vi "UPDATE SETTINGS.vi"(11 "REFERENCES":T1) -> ()   [LabVIEW 2019]
uses:
  Controls/References Cluster.ctl
  Controls/Custom Calendar/Custom Calendar.xctl
  <vilib>/addons/database/Connection.llb/DB Tools Open Connec (String).vi
  <vilib>/addons/database/NI_Database_API.lvlib
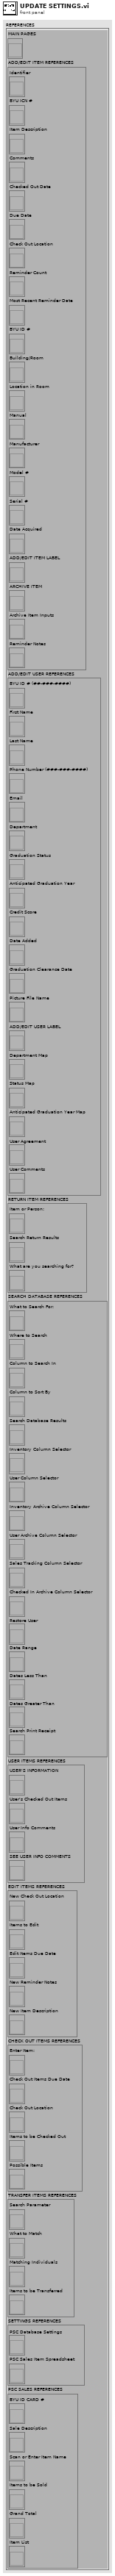
[diagram p1: front panel]
types:
  T1 = typedef "References Cluster.ctl" = cluster{"MAIN PAGES":refnum<vi>, "ADD/EDIT ITEM REFERENCES":cluster{"Identifier":refnum<vi>, "BYU ICN #":refnum<vi>, "Item Description":refnum<vi>, "Comments":refnum<vi>, "Checked Out Date":refnum<vi>, "Due Date":refnum<vi>, "Check Out Location":refnum<vi>, "Reminder Count":refnum<vi>, "Most Recent Reminder Date":refnum<vi>, "BYU ID #":refnum<vi>, "Building/Room":refnum<vi>, "Location in Room":refnum<vi>, "Manual":refnum<vi>, "Manufacturer":refnum<vi>, "Model #":refnum<vi>, "Serial #":refnum<vi>, "Date Acquired":refnum<vi>, "ADD/EDIT ITEM LABEL":refnum<vi>, "ARCHIVE ITEM":refnum<vi>, "Archive Item Inputs":refnum<vi>, "Reminder Notes":refnum<vi>}, "ADD/EDIT USER REFERENCES":cluster{"BYU ID # (##-###-####)":refnum<vi>, "First Name":refnum<vi>, "Last Name":refnum<vi>, "Phone Number (###-###-####)":refnum<vi>, "Email":refnum<vi>, "Department":refnum<vi>, "Graduation Status":refnum<vi>, "Anticipated Graduation Year":refnum<vi>, "Credit Score":refnum<vi>, "Date Added":refnum<vi>, "Graduation Clearance Date":refnum<vi>, "Picture File Name":refnum<vi>, "ADD/EDIT USER LABEL":refnum<vi>, "Department Map":refnum<vi>, "Status Map":refnum<vi>, "Anticipated Graduation Year Map":refnum<vi>, "User Agreement":refnum<vi>, "User Comments":refnum<vi>}, "RETURN ITEM REFERENCES":cluster{"Item or Person:":refnum<vi>, "Search Return Results":refnum<vi>, "What are you searching for?":refnum<vi>}, "SEARCH DATABASE REFERENCES":cluster{"What to Search For:":refnum<vi>, "Where to Search":refnum<vi>, "Column to Search In":refnum<vi>, "Column to Sort By":refnum<vi>, "Search Database Results":refnum<vi>, "Inventory Column Selector":refnum<vi>, "User Column Selector":refnum<vi>, "Inventory Archive Column Selector":refnum<vi>, "User Archive Column Selector":refnum<vi>, "Sales Tracking Column Selector":refnum<vi>, "Checked In Archive Column Selector":refnum<vi>, "Restore User":refnum<vi>, "Date Range":refnum<vi>, "Dates Less Than":refnum<vi>, "Dates Greater Than":refnum<vi>, "Search Print Receipt":refnum<vi>}, "USER ITEMS REFERENCES":cluster{"USER'S INFORMATION":refnum<vi>, "User's Checked Out Items":refnum<vi>, "User Info Comments":refnum<vi>, "SEE USER INFO COMMENTS":refnum<vi>}, "EDIT ITEMS REFERENCES":cluster{"New Check Out Location":refnum<vi>, "Items to Edit":refnum<vi>, "Edit Items Due Date":refnum<vi>, "New Reminder Notes":refnum<vi>, "New Item Description":refnum<vi>}, "CHECK OUT ITEMS REFERENCES":cluster{"Enter Item:":refnum<vi>, "Check Out Items Due Date":refnum<vi>, "Check Out Location":refnum<vi>, "Items to be Checked Out":refnum<vi>, "Possible Items":refnum<vi>}, "TRANSFER ITEMS REFERENCES":cluster{"Search Parameter":refnum<vi>, "What to Match":refnum<vi>, "Matching Individuals":refnum<vi>, "Items to be Transferred":refnum<vi>}, "SETTINGS REFERENCES":cluster{"PSC Database Settings":refnum<vi>, "PSC Sales Item Spreadsheet":refnum<vi>}, "PSC SALES REFERENCES":cluster{"BYU ID CARD #":refnum<vi>, "Sale Description":refnum<vi>, "Scan or Enter Item Name":refnum<vi>, "Items to be Sold":refnum<vi>, "Grand Total":refnum<vi>, "Item List":refnum<vi>}}
  T2 = cluster{"PSC Database Settings":refnum<vi>, "PSC Sales Item Spreadsheet":refnum<vi>}
  T3 = typedef "NI_Database_API.lvlib/Conn ObjectReference.ctl" = refnum<k1>
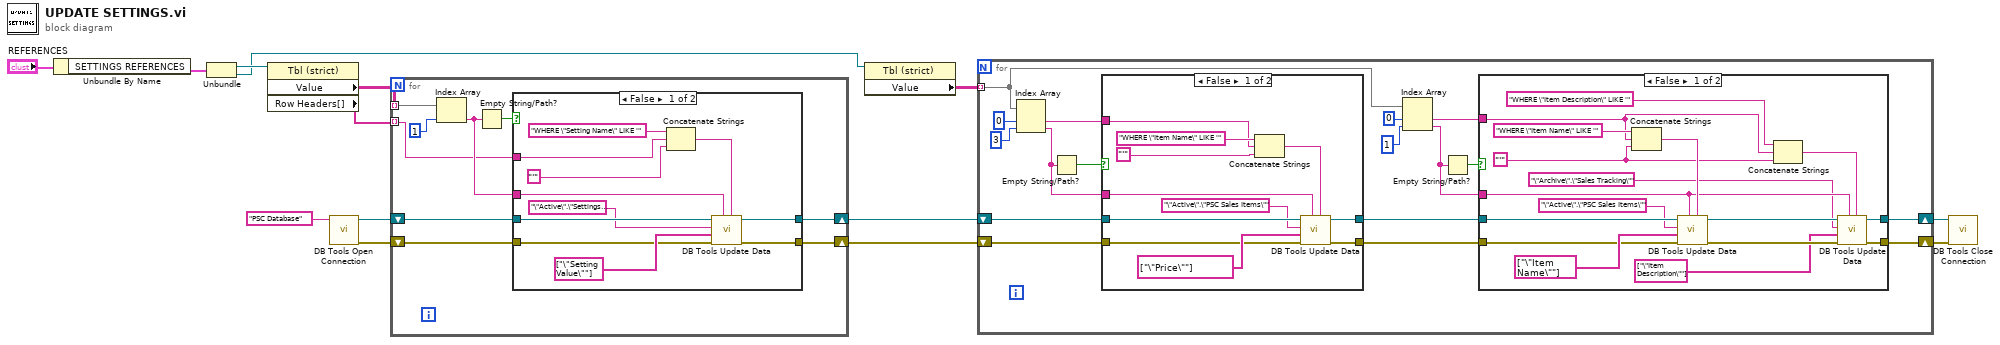
[diagram p0: block diagram]
diagram:
  n1 = Unbundle By Name("REFERENCES") -> ("SETTINGS REFERENCES"=w13:T2)
  n2 = Unbundle(w13) -> ("PSC Database Settings"=w12:refnum<vi>, "PSC Sales Item Spreadsheet"=w6:refnum<vi>)
  n3 = property class="Tbl (strict)"(reference=w12) -> ("Value"=w11:string[][], "Row Headers[]"=w8:string[])  [unwired: 1 in, 2 out]
  n4 = call-poly <vilib>:"DB Tools Open Connection.vi"("connection information"="PSC Database") -> ("error out"=w7:errorcluster, "connection reference"=w9:T3)  [unwired: 7 in]
  n5 = for {
    tunnel: w11 -> [w23] mode=indexing
    shift-right: [w19] -> w4
    shift-left: w9 -> [w20]
    tunnel: w8 -> [w17] mode=indexing
    shift-right: [w15] -> w3
    shift-left: w7 -> [w16]
    n6 = Index Array(array=w23, index=1) -> (element=w18:string)
    n7 = Empty String/Path?(string/path=w18) -> (empty?=w21:bool)
    n8 = case shown="False" w21 {
      tunnel: w20 -> [w34 w36]
      tunnel: [w26 w36] -> w19
      tunnel: w18 -> [w31 _]
      tunnel: w17 -> [w28 _]
      tunnel: w16 -> [w25 w35]
      tunnel: [w24 w35] -> w15
      frame False {
        n9 = Concatenate Strings("WHERE \"Setting Name\" LIKE '", w28, "'") -> (w27:string)
        n10 = call <vilib>:"DB Tools Update Data.vi"("condition"=w27, "data"=w31, "error in (no error)"=w25, "columns"=string[] ["\"Setting Value\""], "table"="\"Active\".\"Settings\"", "connection reference"=w34) -> ("error out"=w24:errorcluster, "connection reference out"=w26:T3)  [unwired: 4 in]
      }
      frame True {
      }
    }
  }
  n11 = property class="Tbl (strict)"(reference=w6) -> ("Value"=w5:string[][])  [unwired: 1 in, 2 out]
  n12 = for {
    tunnel: w5 -> [w41] mode=indexing
    shift-right: [w38] -> w2
    shift-left: w4 -> [w43]
    shift-right: [w37] -> w1
    shift-left: w3 -> [w42]
    n13 = Index Array(array=w41, index #1=0 ("index"), index #2=3 ("index")) -> (element #1=w44:string, element #2=w45:string)
    n14 = Empty String/Path?(string/path=w45) -> (empty?=w46:bool)
    n15 = case shown="False" w46 {
      tunnel: w43 -> [w64 w66]
      tunnel: [w55 w66] -> w40
      tunnel: w45 -> [w58 _]
      tunnel: w42 -> [w59 w65]
      tunnel: [w54 w65] -> w39
      tunnel: w44 -> [w57 _]
      frame False {
        n16 = Concatenate Strings("WHERE \"Item Name\" LIKE '", w57, "'") -> (w60:string)
        n17 = call <vilib>:"DB Tools Update Data.vi"("condition"=w60, "data"=w58, "error in (no error)"=w59, "columns"=string[] ["\"Price\""], "table"="\"Active\".\"PSC Sales Items\"", "connection reference"=w64) -> ("error out"=w54:errorcluster, "connection reference out"=w55:T3)  [unwired: 4 in]
      }
      frame True {
      }
    }
    n18 = Index Array(array=w41, index #1=0 ("index"), index #2=1 ("index")) -> (element #1=w49:string, element #2=w50:string)
    n19 = Empty String/Path?(string/path=w50) -> (empty?=w52:bool)
    n20 = case shown="False" w52 {
      tunnel: w40 -> [w83 w85]
      tunnel: [w68 w85] -> w38
      tunnel: w50 -> [w75 _]
      tunnel: w39 -> [w78 w84]
      tunnel: [w67 w84] -> w37
      tunnel: w49 -> [w71 _]
      frame False {
        w70 = "'"
        n21 = Concatenate Strings("WHERE \"Item Name\" LIKE '", w71, w70) -> (w79:string)
        n22 = call <vilib>:"DB Tools Update Data.vi"("condition"=w79, "data"=w75, "error in (no error)"=w78, "columns"=string[] ["\"Item Name\""], "table"="\"Active\".\"PSC Sales Items\"", "connection reference"=w83) -> ("error out"=w76:errorcluster, "connection reference out"=w77:T3)  [unwired: 4 in]
        n23 = Concatenate Strings("WHERE \"Item Description\" LIKE '", w71, w70) -> (w69:string)
        n24 = call <vilib>:"DB Tools Update Data.vi"("condition"=w69, "data"=w75, "error in (no error)"=w76, "columns"=string[] ["\"Item Description\""], "table"="\"Archive\".\"Sales Tracking\"", "connection reference"=w77) -> ("error out"=w67:errorcluster, "connection reference out"=w68:T3)  [unwired: 4 in]
      }
      frame True {
      }
    }
  }
  n25 = call <vilib>:"DB Tools Close Connection.vi"("error in (no error)"=w1, "connection reference"=w2) -> ()  [unwired: 5 in, 1 out]
